vi "Configure Trigger Level.vi"(8 "error in (no error)":errorcluster, 9 "Trigger Type":u16(ring) items=["Edge", "Pulse", "TV", "Pattern"], 10 "Trigger Level (0.0 V)":dbl, 11 "VISA resource name":refnum<visa-resource-name>) -> (0 "error out":errorcluster, 3 "VISA resource name out":refnum<visa-resource-name>)   [LabVIEW 2010, in "Agilent DSO1000 Series.lvlib"]
doc: "This VI configures trigger level."
uses:
  <instrlib>/Agilent DSO1000 Series/Agilent DSO1000 Series.lvlib
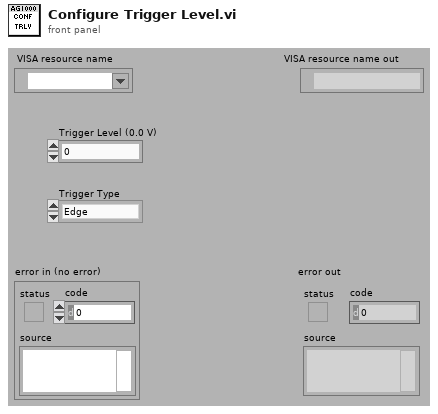
[diagram p1: front panel]
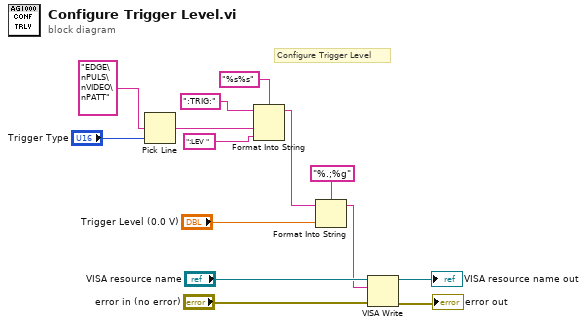
[diagram p0: block diagram]
diagram:
  # "Configure Trigger Level"
  n1 = Pick Line(multi-line string="EDGE\nPULS\nVIDEO\nPATT", line index="Trigger Type") -> (output string=w4:string)  [unwired: 1 in]
  n2 = Format Into String(format string="%s%s", initial string=":TRIG:", w4, ":LEV ") -> (resulting string=w3:string)  [unwired: 1 in, 1 out]
  n3 = Format Into String(format string="%.;%g", initial string=w3, "Trigger Level (0.0 V)") -> (resulting string=w9:string)  [unwired: 1 in, 1 out]
  n4 = VISA Write(VISA resource name="VISA resource name", write buffer=w9, error in (no error)="error in (no error)") -> (VISA resource name out=→"VISA resource name out":refnum<visa-resource-name>, error out=→"error out":errorcluster)  [unwired: 1 out]
